vi "web test v4.vi"() -> ()   [LabVIEW 2013]
uses:
  <vilib>/Platform/TimedLoop/XDataNode/timing_clust.ctl
  <vilib>/Platform/TimedLoop/XDataNode/nitl_modes.ctl
  <vilib>/Platform/TimedLoop/XDataNode/wakeup.ctl
  Web test/Global 1.vi
  <vilib>/platform/TimedLoop/XDataNode/XDataNode.xnode
  <vilib>/Platform/TimedLoop/XDataNode/XDNodeRunTimeDep.lvlib
panel:
  in  "Stop Disp":bool
  in  "Tab Control":enum32{"Page 1", "Page 2", "Page 3"}(tab)
  out "X1":dbl
  out "X5":dbl
  out "Boolean":bool
  in  "Stop All":bool
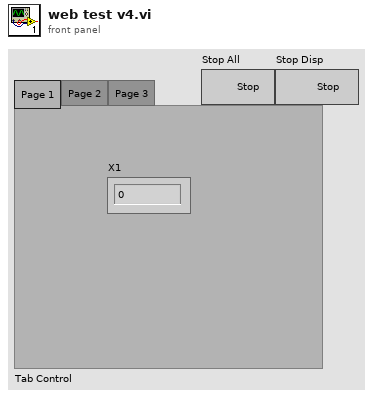
[diagram p1: front panel]
types:
  T1 = typedef "XDNodeRunTimeDep.lvlib/timing_clust.ctl" = cluster{"Expected End [f-1]":u64, "Actual End [f-1]":u64, "Finished Late? [f-1]":bool, "Expected End [i-1]":u64, "Actual End [i-1]":u64, "Finished Late? [i-1]":bool, "Expected Start [i]":u64, "Actual Start [i]":u64, "Expected Start [f]":u64, "Actual Start [f]":u64, "Source Name":string, "Structure Name":string, "Period":i64, "Deadline":i64, "Offset":i64, "Start":i64, "Priority":i32, "Timeout":i32, "Mode":T2, "Wakeup Reason":T3, "Error":errorcluster, "Source Type":string, "Secondary Source Type":string, "Global End Time":u64, "Global Start Time":u64, "Frame Duration":u64, "Iteration Duration":u64, "Assigned CPU":i32, "I/O Scan Engine Mode":u32}
  T2 = typedef "XDNodeRunTimeDep.lvlib/nitl_modes.ctl" = enum32{"No Change", "Process missed periods, maintain original phase", "Discard missed periods, maintain original phase", "Process missed periods, ignore original phase", "Discard missed periods, ignore original phase"}
  T3 = typedef "XDNodeRunTimeDep.lvlib/wakeup.ctl" = enum32{"Normal", "Aborted", "Asynchronous wakeup", "Timing source error", "Timed loop error", "Timeout"}
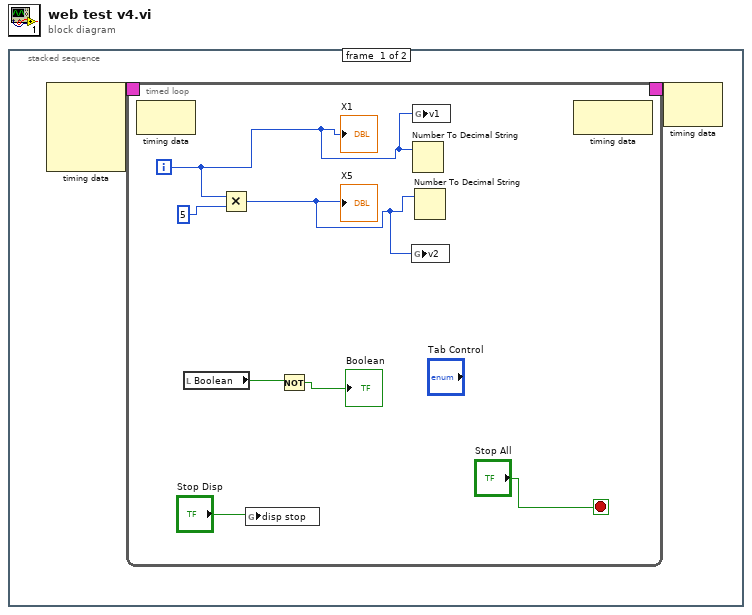
[diagram p0: block diagram]
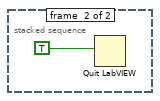
[diagram p2: hidden frame]
diagram:
  n1 = stacked-sequence {
    frame #0 {
      n2 = node-c288() -> (w2:T1)  [unwired: 4 in]
      n3 = timed-loop {
        timing: w2 -> [_]
        timing-out: [_] -> w1
        i -> [w6]
        stop <- "Stop All" stop-if-true
        n4 = node-c288() -> ()  [unwired: 1 in, 1 out]
        n5 = local read "Boolean"() -> (w8:bool)
        n6 = Multiply(x=w6, y=5) -> (x*y=w5:i32)
        "X5" <- w5
        n7 = global write "Global 1.vi" "disp stop"("Stop Disp") -> ()
        n8 = Not(x=w8) -> (.not. x?=→"Boolean":bool)
        n9 = global write "Global 1.vi" "v2"(w5) -> ()
        n10 = global write "Global 1.vi" "v1"(w6) -> ()
        n11 = Number To Decimal String(number=w6) -> ()  [unwired: 1 in, 1 out]
        n12 = Number To Decimal String(number=w5) -> ()  [unwired: 1 in, 1 out]
        n13 = node-c288() -> ()  [unwired: 1 in, 1 out]
        "X1" <- w6
      }
      n14 = node-c288(w1) -> ()  [unwired: 1 out]
    }
    frame #1 {
      n15 = Quit LabVIEW(quit? (T)=TRUE) -> ()
    }
  }
